vi "Get Channel Labels.vi"(9 "error in (no error)":errorcluster, 10 "Configuration":T1, 11 "Corvus Byte Datatype in":refnum<class "Corvus Byte Datatype.lvclass">) -> (1 "error out":errorcluster, 2 "Channel Label(s)":string[](array[string]), 3 "Corvus Byte Datatype out":refnum<class "Corvus Byte Datatype.lvclass">)   [LabVIEW 2021, in "Corvus Byte Datatype.lvclass"]
uses:
  Corvus Byte Datatype.lvclass
  <userlib>/S2 Labs/Modbus Toolkit/TypeDefs/MB Element.ctl
  <userlib>/S2 Labs/Modbus Toolkit/TypeDefs/Endianness Type.ctl
  <userlib>/S2 Labs/Modbus Toolkit/TypeDefs/Access Type.ctl
  Corvus Byte Datatype.lvclass/Corvus Byte Datatype.ctl
  <userlib>/S2 Labs/Modbus Toolkit/S2L Modbus API.lvclass
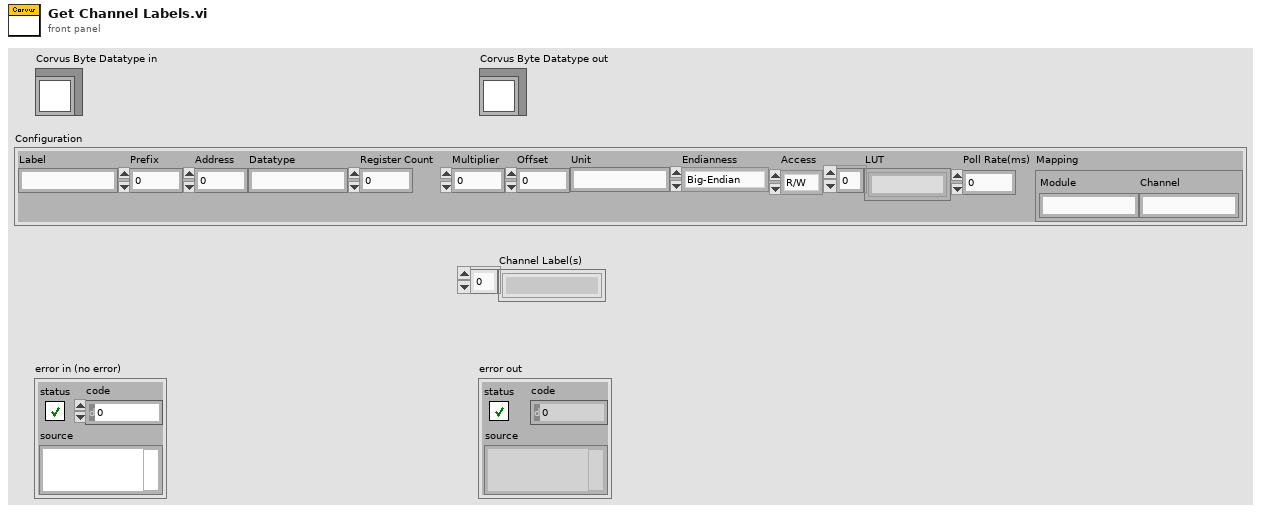
[diagram p1: front panel]
types:
  T1 = typedef "S2L Modbus API.lvclass/MB Element.ctl" = cluster{"Label":string, "Prefix":u8, "Address":u16, "Datatype":string, "Register Count":u8, "Multiplier":dbl, "Offset":dbl, "Unit":string, "Endianness":T2, "Access":T3, "LUT":string[], "Poll Rate(ms)":u16, "Mapping":cluster{"Module":string, "Channel":string}}
  T2 = typedef "Endianness Type.ctl" = enum16{"Big-Endian", "Little-Endian", "Big-Endian Byte Swap", "Little-Endian Byte Swap"}
  T3 = typedef "S2L Modbus API.lvclass/Access Type.ctl" = enum16{"R/W", "R", "W"}
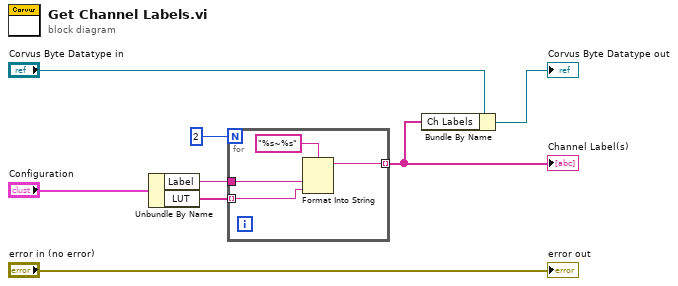
[diagram p0: block diagram]
diagram:
  n1 = Unbundle By Name("Configuration") -> ("Label"=w6:string, "LUT"=w5:string[])
  n2 = for {
    N: 2 -> [_]
    tunnel: w6 -> [w11]
    tunnel: w5 -> [w10] mode=indexing
    tunnel: [w9] -> w1 mode=indexing
    n3 = Format Into String(format string="%s~%s", w11, w10) -> (resulting string=w9:string)  [unwired: 2 in, 1 out]
  }
  "Channel Label(s)" <- w1
  n4 = Bundle By Name(cluster="Corvus Byte Datatype in", "Ch Labels"=w1) -> (→"Corvus Byte Datatype out":refnum<class "Corvus Byte Datatype.lvclass">)
  "error out" <- "error in (no error)"
